vi "Insert CVT Data.vi"(7 "Group":string, 8 "error in":errorcluster, 9 "Data":variant, 10 "tag":string, 11 "cvt in":variant) -> (0 "error out":errorcluster, 3 "cvt out":variant)   [LabVIEW 2014, in "CVT.lvclass"]
uses:
  CVT.lvclass
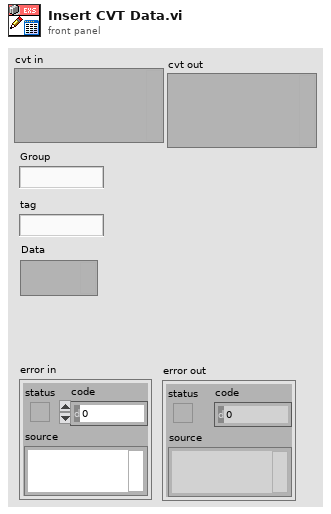
[diagram p1: front panel]
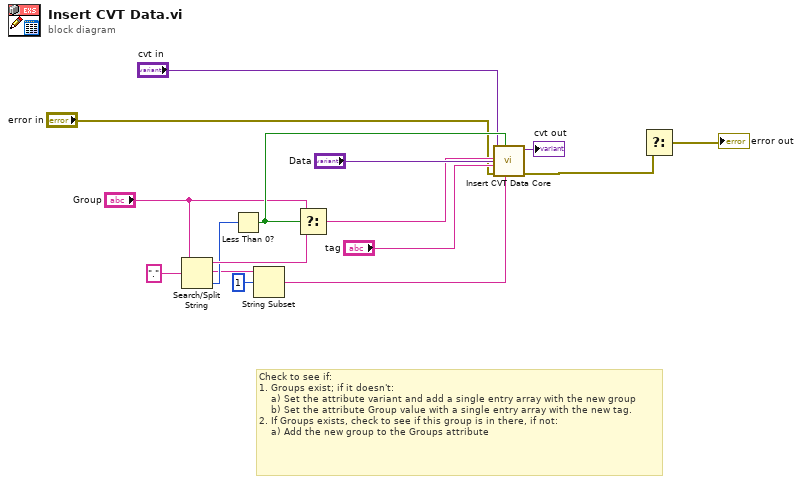
[diagram p0: block diagram]
diagram:
  # "Check to see if:\n1. Groups exist; if it doesn't:\n    a) Set the attribute variant and add a single entry array with the new group\n    b) Set the attribute Group value with a single entry array with the new tag.\n2. If Groups exists, check to see if this group is in there, if not:\n    a) Add the new group to the Groups attribute"
  n1 = Search/Split String(string="Group", search string/char (-)="." ("regular expression")) -> (substring before match=w10:string, match + rest of string=w6:string, offset of match=w9:i32)  [unwired: 1 in]
  n2 = Less Than 0?(x=w9) -> (x < 0?=w11:bool)
  n3 = String Subset(string=w6, offset (0)=1) -> (substring=w4:string)  [unwired: 1 in]
  n4 = Select(t="Group", s=w11, f=w10) -> (s? t:f=w12:string)
  n5 = call "Insert CVT Data Core.vi"("Data"="Data", "Nested Group"=w4, "Nested?"=w11, "error in (no error)"="error in", "tag"="tag", "Group"=w12, "CVT In"="cvt in") -> ("error out"=w14:errorcluster, "CVT Out"=→"cvt out":variant)  [unwired: 2 in]
  n6 = Select(f=w14) -> (s? t:f=→"error out":errorcluster)  [unwired: 2 in]
